vi "scani_test.vi"() -> ()   [LabVIEW 2019]
panel:
  out "error out":errorcluster
  out "Scanivalve Pressures":cluster{i32[], "Array":dbl[]}(graph)={[1, 2, 3, 4, 5, 6, 7, 8, 9, 10, 11, 12, 13, 14, 15, 16], "Array"=[107.2386417388916, 109.67449417114258, 112.26835975646972, 113.32290878295899, 113.25851020812988, 110.12275047302246, 110.01677665710449, 110.23803977966308, 111.38681907653809, 112.57089157104492, 115.55567054748535, 109.39623069763184, 115.34736213684081, 113.26969871520996, 112.33615150451661, 111.57799453735352]}
  in  "stop":bool
  in  "Samples per Set to Save(Set before running)":dbl=20.0 caption="Samples per Set to Save" min=1.0 max=500.0 step=1.0 format="%#_13g"
  out "Sampling Rate":dbl=500.0
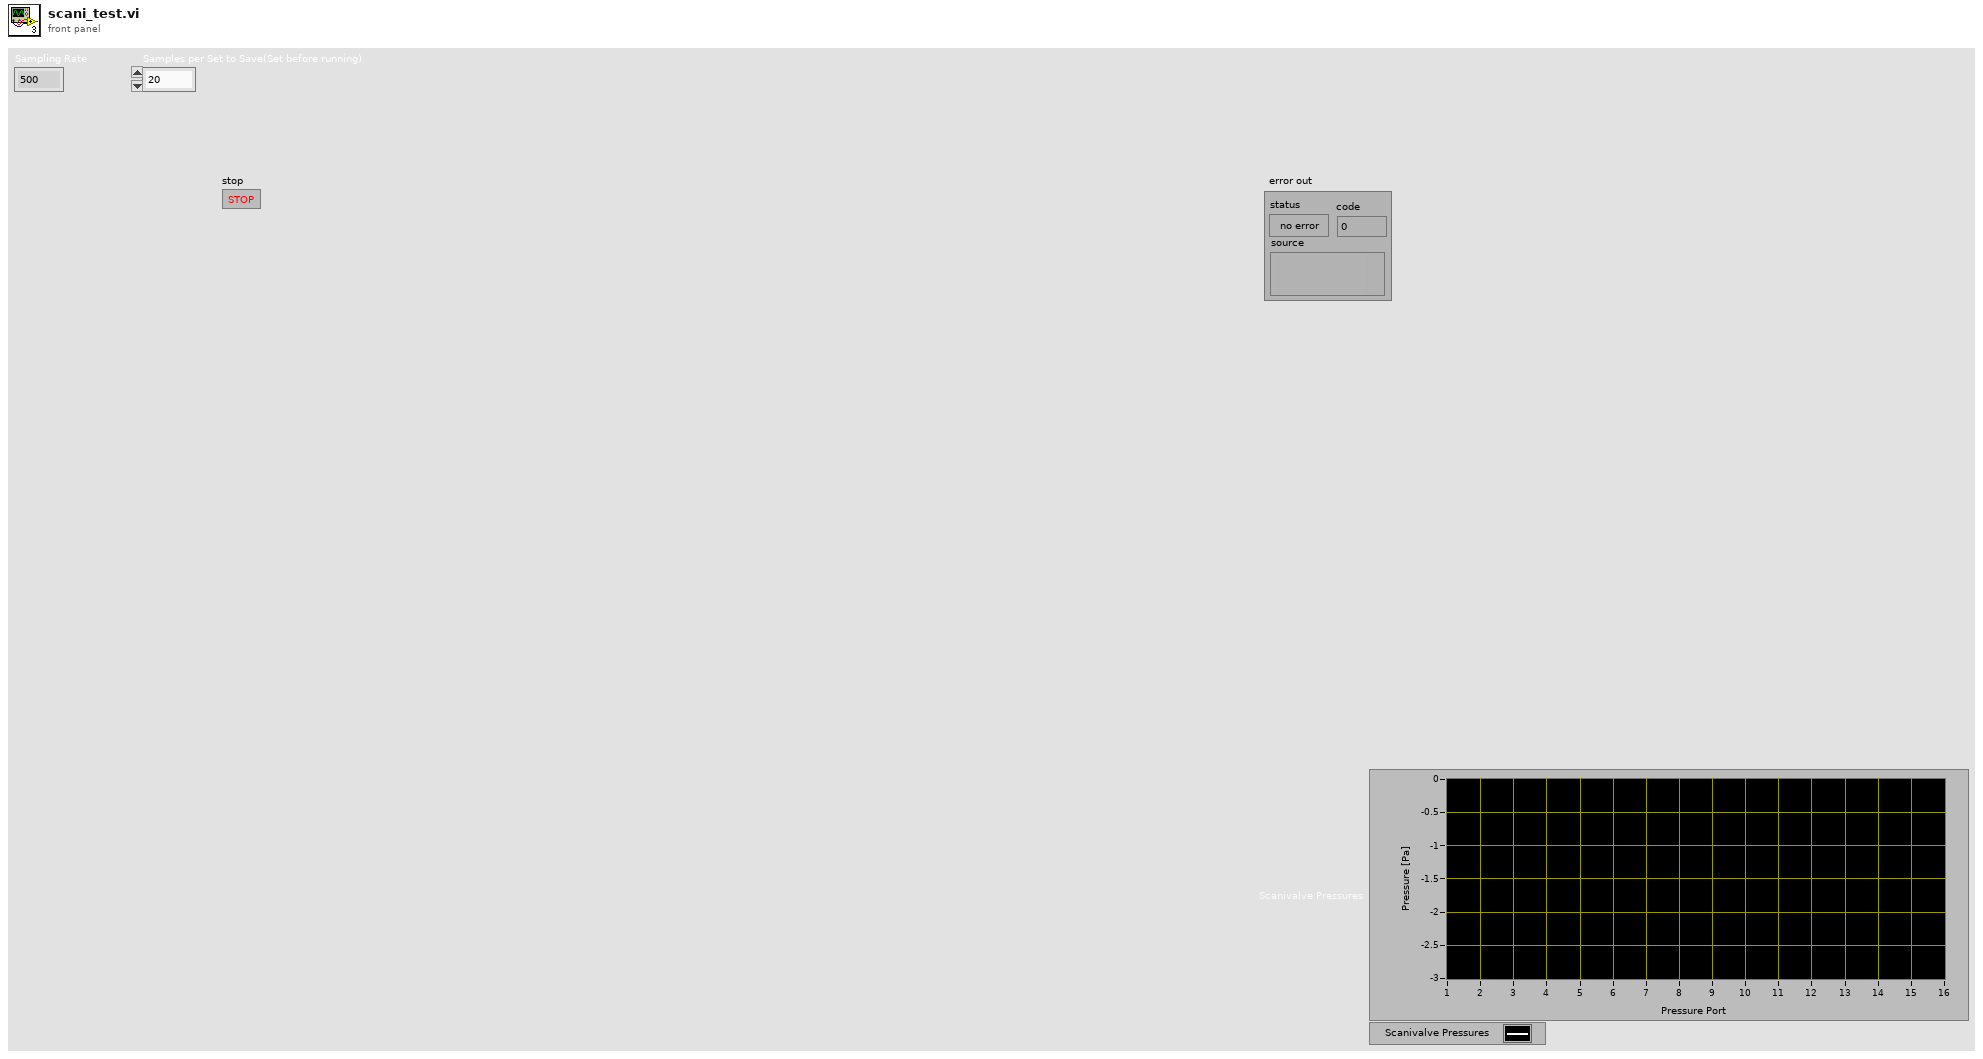
[diagram p1: front panel]
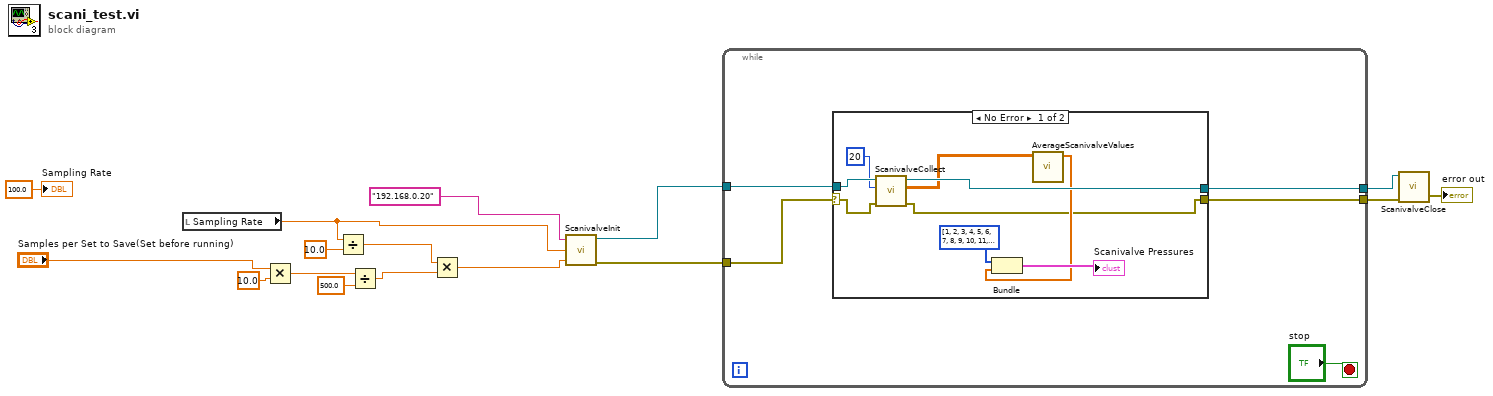
[diagram p0: block diagram]
diagram:
  n1 = local read "Sampling Rate"() -> (w7:dbl)
  n2 = Multiply(x="Samples per Set to Save(Set before running)", y=10.0) -> (x*y=w15:dbl)
  n3 = Divide(x=w7, y=10.0) -> (x/y=w11:dbl)
  n4 = Divide(x=w15, y=500.0) -> (x/y=w10:dbl)
  n5 = Multiply(x=w11, y=w10) -> (x*y=w6:dbl)
  n6 = call "ScanivalveInit.vi"("Scanner IP Address"="192.168.0.20", "Sampling Frequency Requested (Hz)"=w7, "Total # of Samples to Collect"=w6) -> ("TCP Network Connection out"=w4:refnum<k5>, "error out"=w5:errorcluster)  [unwired: 2 in]
  n7 = while {
    tunnel: w5 -> [w20]
    tunnel: w4 -> [w19]
    tunnel: [w18] -> w3
    tunnel: [w17] -> w2
    stop <- "stop" stop-if-true
    n8 = case shown="No Error" w20 {
      selector: w20 -> [w23 w31]
      tunnel: w19 -> [w30 w32]
      tunnel: [w29 w32] -> w18
      tunnel: [w22 w31] -> w17
      frame No Error {
        n9 = call "ScanivalveCollect.vi"("error in (no error)"=w23, "Samples per query."=20, "connection ID"=w30) -> ("error out"=w22:errorcluster, "Px Array"=w28:sgl[][], "connection ID out"=w29:refnum<k5>)  [unwired: 1 in, 1 out]
        n10 = call "AverageScanivalveValues.vi"("Px Array"=w28) -> ("Array"=w25:dbl[])  [unwired: 10 in]
        n11 = Bundle(i32[] [1, 2, 3, 4, 5, 6, 7, 8, 9, 10, 11, 12, 13, 14, 15, 16], "Array"=w25) -> (→"Scanivalve Pressures":cluster{i32[], "Array":dbl[]})  [unwired: 1 in]
      }
      frame Error {
      }
    }
  }
  n12 = call "ScanivalveClose.vi"("error in (no error)"=w2, "connection ID"=w3) -> ("error out"=→"error out":errorcluster)  [unwired: 3 in]
  "Sampling Rate" <- 100.0 ("Sampling Rate")
